vi "Get_IP_Number.vi"() -> (0 "IP Number":string)   [LabVIEW 2011]
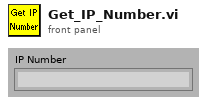
[diagram p1: front panel]
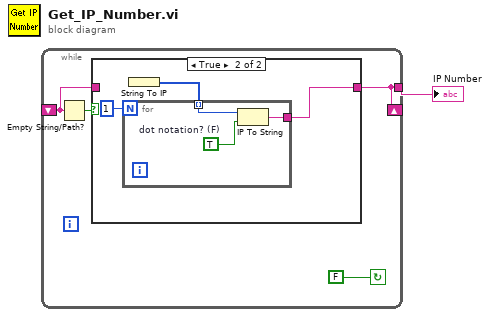
[diagram p0: block diagram]
diagram:
  n1 = while {
    shift-left: _ -> [w3]
    shift-right: [w5] -> _
    tunnel: [w5] -> w1
    stop <- FALSE continue-if-true
    n2 = Empty String/Path?(string/path=w3) -> (empty?=w4:bool)
    n3 = case shown="True" w4 {
      tunnel: [w6 w8] -> w5
      tunnel: w3 -> [w6 _]
      frame False {
      }
      frame True {
        n4 = String To IP() -> (0:w9:u32[])  [unwired: 1 out]
        n5 = for {
          N: 1 -> [_]
          tunnel: w9 -> [w12] mode=indexing
          tunnel: [w11] -> w8
          w10 = TRUE  # dot notation? (F)
          n6 = IP To String(1:w10, 2:w12) -> (0:w11:string)
        }
      }
    }
  }
  "IP Number" <- w1
